vi "Get DoubleArray.vi"(8 "error in (no error)":errorcluster, 11 "DoubleArrayMsg In":refnum<class "DoubleArrayMsg.lvclass">) -> (0 "error out":errorcluster, 2 "Message Data":dbl[](array[numeric]), 3 "DoubleArrayMsg Out":refnum<class "DoubleArrayMsg.lvclass">)   [LabVIEW 2017, in "LapDog.Messaging.v3.NativeArrays.lvlib" / "DoubleArrayMsg.lvclass"]
doc: "Returns the data contained in the message.\n\nThis method executes regardless of the error in state."
uses:
  DoubleArrayMsg.lvclass
  DoubleArrayMsg.lvclass/DoubleArrayMsg.ctl
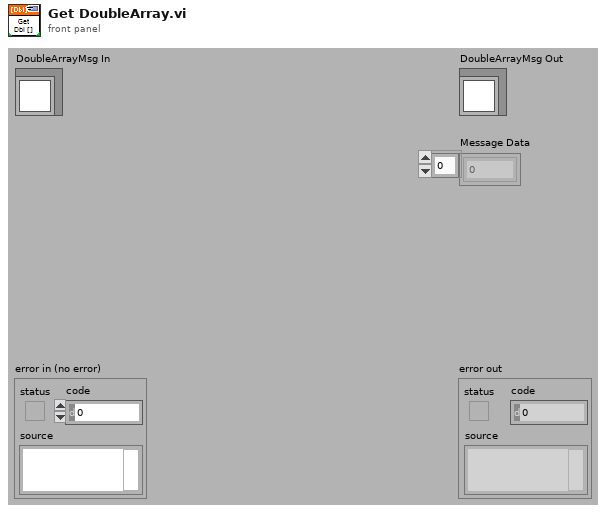
[diagram p1: front panel]
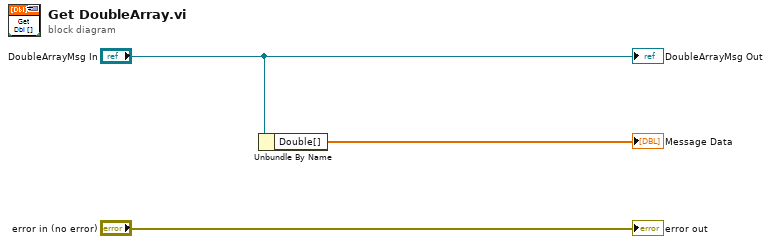
[diagram p0: block diagram]
diagram:
  n1 = Unbundle By Name("DoubleArrayMsg In") -> ("Double[]"=→"Message Data":dbl[])
  "error out" <- "error in (no error)"
  "DoubleArrayMsg Out" <- "DoubleArrayMsg In"
